vi "Teleop.vi"(10 "Match Info":T1={"Autonomous Elapsed Seconds"=0.0, "TeleOp Elapsed Seconds"=62.077, "Disabled Elapsed Seconds"=2.193, "Visited Autonomous"=FALSE, "Visited TeleOp"=TRUE, "Visited Disabled"=TRUE, "Autonomous Settings"={"Autonomous Style"=enum."Independent", "VI Refnum"=refnum}}, 11 "Call Context":T2=enum."Stop") -> ()   [LabVIEW 2016]
doc: "This VI is called for each TeleOp packet received from the DS where the robot is not disabled. It is often used to read from the joysticks and update I/O or to update setpoints for timed control loops. It should complete and return within 20 milliseconds or it may miss DS packets."
uses:
  <vilib>/Rock Robotics/WPI/DriverStation/WPI_DriverStationDerivedRobotMode.ctl
  <vilib>/Rock Robotics/WPI/DriverStation/WPI_DriverStationMatch Info.ctl
  Typedef/XBox Axis.ctl
  Typedef/XBox Buttons.ctl
  <vilib>/Rock Robotics/WPI/Solenoid/WPI_SolenoidValue.ctl
  <vilib>/Rock Robotics/WPI/Utilities/WPI_GetSetVariantRefNum.vi
  <vilib>/Rock Robotics/Network Tables/NT Write Boolean Array.vi
  <vilib>/Rock Robotics/Network Tables/NT Write Numeric Array.vi
  <vilib>/Rock Robotics/WPI/Solenoid/WPI_SolenoidSetEnum.vi
  SubSystems/Drive/Drive System.lvlib
  SubSystems/Intake/Intake.lvlib
  Vision/Vision Drive/Vision Drive.lvlib
panel:
  in  "Y Motor Deadbnd":dbl(slide)=0.5510204081632653 scale=0.0..1.0
  in  "X Motor Deadbnd":dbl(slide)=0.6836734693877551 scale=0.0..1.0
  in  "Y max power":dbl(slide)=0.7244897959183673 scale=0.0..1.0
  in  "X max power":dbl(slide)=0.6326530612244897 scale=0.0..1.0
  in  "Y sensitivity 2":dbl(slide)=1.0 scale=0.0..1.0
  in  "X sensitivity 2":dbl(slide)=0.2857142857142857 scale=0.0..1.0
  in  "X Joy Dead":dbl=0.06
  in  "Y Joy Dead":dbl=0.08
  out "Angle":dbl
  in  "Reset Gyro":bool
  in  "Value":bool
  in  "Setting":enum16{"Custom", "Boiler", "Gear"}(ring)
  in  "Custom":i32
  in  "X sensitivity":dbl(slide) scale=0.0..1.0
  in  "X deadband":dbl=0.3
  in  "Y sensitivity":dbl(slide)=1.0 scale=0.0..1.0
  in  "Y deadband":dbl=0.38
  # "Normal Mode"
  # "Climb Mode"
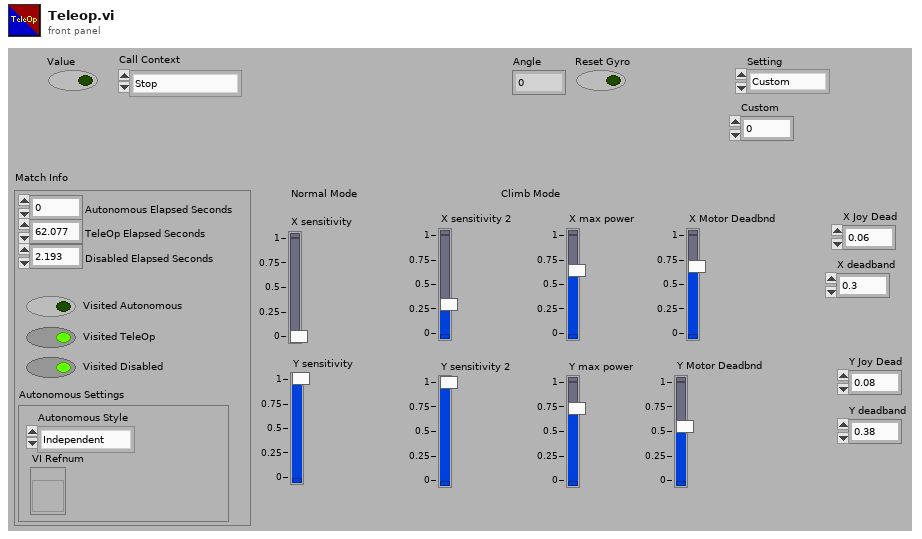
[diagram p1: front panel]
types:
  T1 = typedef "WPI_DriverStationMatch Info.ctl" = cluster{"Autonomous Elapsed Seconds":dbl, "TeleOp Elapsed Seconds":dbl, "Disabled Elapsed Seconds":dbl, "Visited Autonomous":bool, "Visited TeleOp":bool, "Visited Disabled":bool, "Autonomous Settings":cluster{"Autonomous Style":enum16{"Iterative", "Independent"}, "VI Refnum":refnum<vi>}}
  T2 = typedef "WPI_DriverStationDerivedRobotMode.ctl" = enum16{"Init", "Execute", "Stop"}
  T3 = typedef "XBox Buttons.ctl" = enum16{"A", "B", "X", "Y", "Left Bumper", "Right Bumper", "Back", "Start", "Left Joystick", "Right Joystick"}
  T4 = typedef "XBox Axis.ctl" = enum16{"Left X", "Left Y", "Left Trigger", "Right Trigger", "Right X", "Right Y"}
  T5 = typedef "WPI_JoystickDevRef.ctl" = cluster{"Device":T6}
  T6 = typedef "WPI_JoystickDeviceEnum.ctl" = enum16{"USB 0", "USB 1", "USB 2", "USB 3", "USB 4", "USB 5"}
  T7 = typedef "WPI_GyroDevRef.ctl" = cluster{"DevStatus":errorcluster, "Analog Channel":T8, "Offset":dbl, "Gain (VoltsPerDegree/Second)":dbl, "Gyro Type":enum16{"Analog", "XRS450"}, "Handle":i32, "SPI Bus":T9, "Device Found":bool, "Sample Rate":dbl, "Calibrate On Open":bool}
  T8 = typedef "FPGA_AIChannel.ctl" = enum8{"AI 0", "AI 1", "AI 2", "AI 3", "AI MXP 0", "AI MXP 1", "AI MXP 2", "AI MXP 3", "Invalid"}
  T9 = typedef "spi_bus.ctl" = enum16{"SPI On-Board, CS0", "SPI On-Board, CS1", "SPI On-Board, CS2", "SPI On-Board, CS3", "SPI MXP", "Invalid"}
  T10 = typedef "WPI_MotorControlDeviceRef.ctl" = cluster{"DeviceStatus":errorcluster, "Type":T11, "PWM":cluster{"PWM Channel":T12, "DeadBand":T13}, "CAN":cluster{"Device Number":u8, "SetOutput VI Ref":variant, "GetOutput VI Ref":variant, "Enable VI Ref":variant, "Disable VI Ref":variant, "Data":variant}, "Invert":bool}
  T11 = typedef "WPI_MotorControlType.ctl" = enum16{"PWM", "CAN"}
  T12 = typedef "FPGA_DIOPWMChannel.ctl" = enum8{"PWM 0", "PWM 1", "PWM 2", "PWM 3", "PWM 4", "PWM 5", "PWM 6", "PWM 7", "PWM 8", "PWM 9", "PWM MXP 0", "PWM MXP 1", "PWM MXP 2", "PWM MXP 3", "PWM MXP 4", "PWM MXP 5", "PWM MXP 6", "PWM MXP 7", "PWM MXP 8", "PWM MXP 9", "Invalid"}
  T13 = typedef "WPI_PWMDeadband.ctl" = cluster{"Name":string, "maxPositivePwm":i32, "minPositivePwm":i32, "centerPwm":i32, "maxNegativePwm":i32, "minNegativePwm":i32, "angularRange":u16}
  T14 = typedef "WPI_SolenoidValue.ctl" = enum16{"Off", "On", "Forward", "Reverse"}
  T15 = typedef "WPI_SolenoidDevRef.ctl" = cluster{"DevStatus":errorcluster, "Pneumatics Control Module":u8, "Forward Solenoid Channel":T16, "Reverse Solenoid Channel":T16}
  T16 = typedef "WPI_SolenoidChannel.ctl" = enum8{"Solenoid 0", "Solenoid 1", "Solenoid 2", "Solenoid 3", "Solenoid 4", "Solenoid 5", "Solenoid 6", "Solenoid 7", "Invalid"}
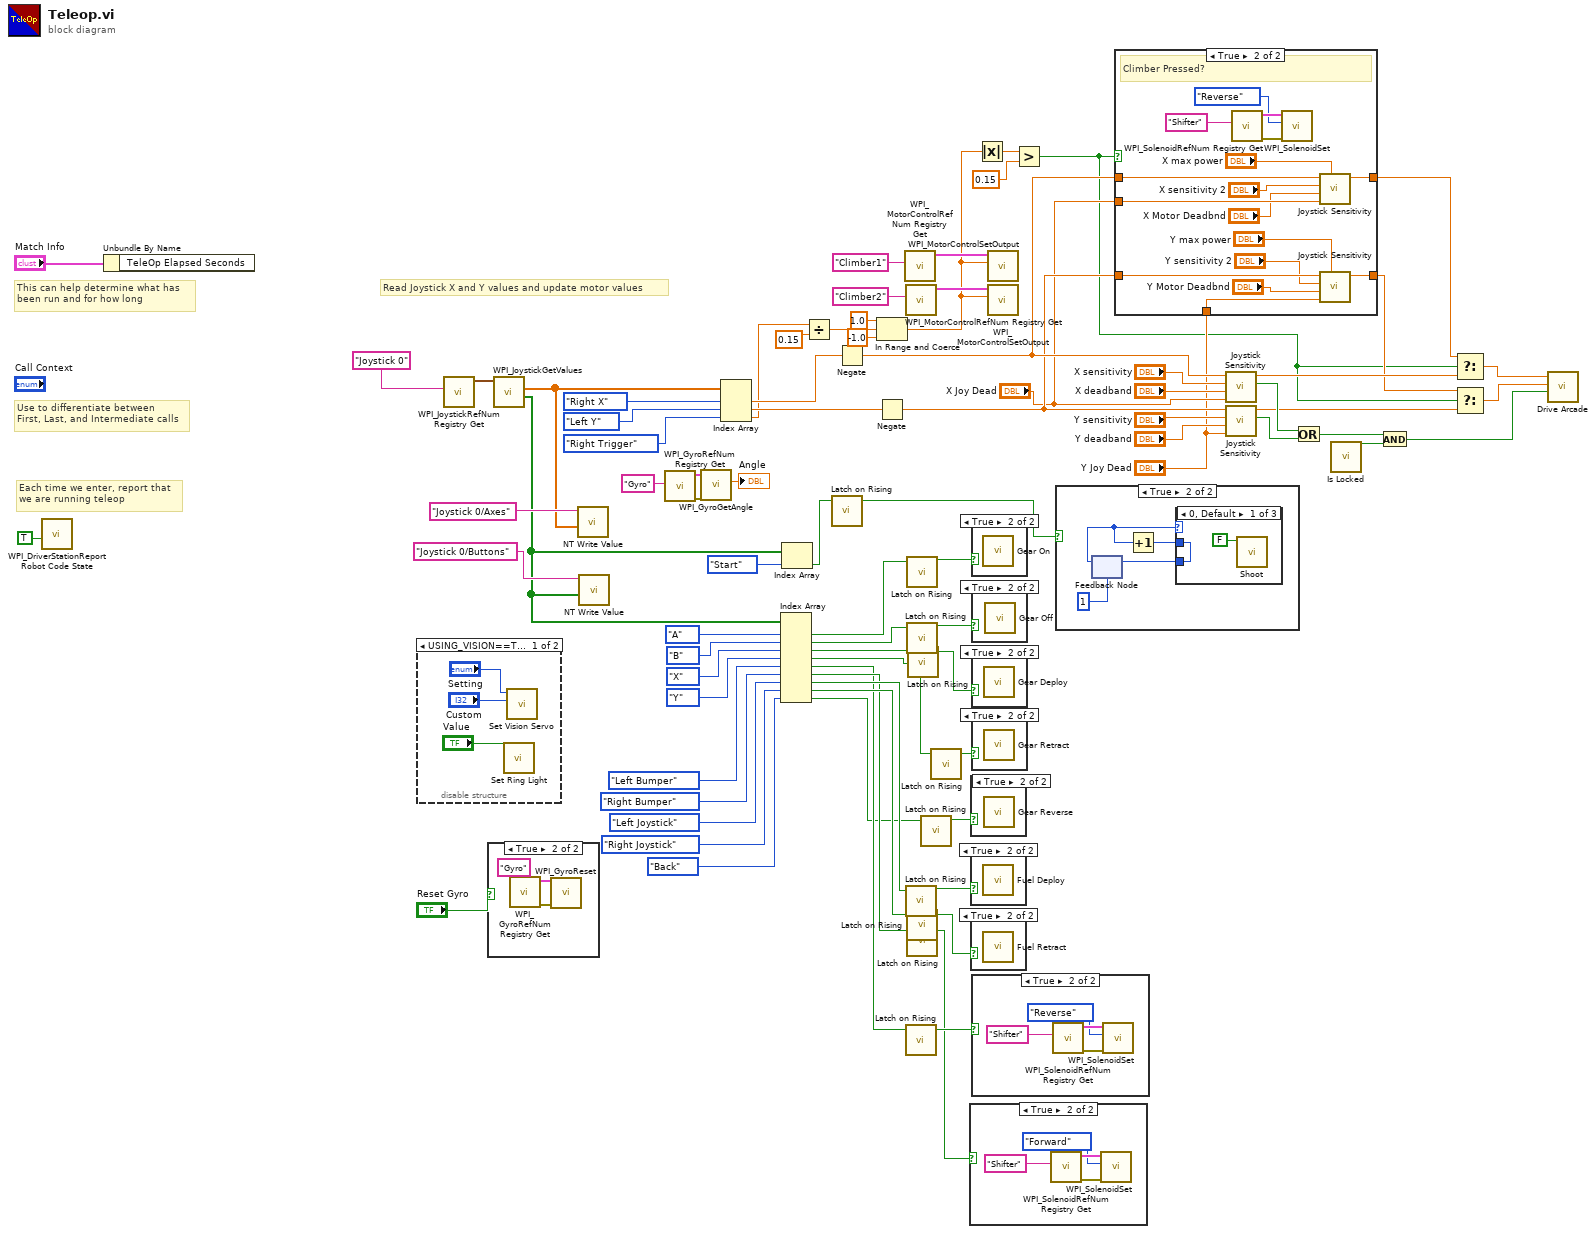
[diagram p0: block diagram]
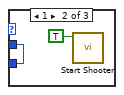
[diagram p5: hidden frame]
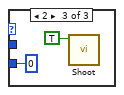
[diagram p6: hidden frame]
diagram:
  # "Each time we enter, report that\nwe are running teleop"
  # "Use to differentiate between\nFirst, Last, and Intermediate calls"
  # "This can help determine what has\nbeen run and for how long"
  # "Read Joystick X and Y values and update motor values"
  n1 = call <vilib>:"WPI_DriverStationReport Robot Code State.vi"("TeleOp"=TRUE ("Autonomous")) -> ()  [unwired: 10 in, 1 out]
  n2 = Unbundle By Name("Match Info") -> ()  [unwired: 1 out]
  n3 = disable-structure shown="USING_VISION==TRUE" {
    frame condition #0 (active) {
      n4 = call "Set Ring Light.vi"("Light On? (F)"="Value") -> ()  [unwired: 10 in, 1 out]
      n5 = call "Set Vision Servo.vi"("Custom"="Custom", "Setting"="Setting") -> ()  [unwired: 9 in, 1 out]
    }
    frame condition #1 {
    }
  }
  n6 = call <vilib>:"WPI_JoystickRefNum Registry Get.vi"("refnum name"="Joystick 0") -> ("JoystickDevRef"=w78:T5)  [unwired: 1 in, 9 out]
  n7 = case shown="True" "Reset Gyro" {
    frame False {
    }
    frame True {
      n8 = call <vilib>:"WPI_GyroRefNum Registry Get.vi"("refnum name"="Gyro") -> ("error out"=w86:errorcluster, "GyroDevRef"=w85:T7)  [unwired: 9 in]
      n9 = call <vilib>:"WPI_GyroReset.vi"("error in"=w86, "GyroDevRef"=w85) -> ()  [unwired: 8 in, 2 out]
    }
  }
  n10 = call <vilib>:"WPI_JoystickGetValues.vi"("JoystickDevRef"=w78) -> ("Buttons"=w33:bool[], "Axes"=w74:dbl[])  [unwired: 6 in, 3 out]
  n11 = call-poly <vilib>:"NT Write Value.vi"("Numeric Array"=w74, "Name"="Joystick 0/Axes") -> ()  [unwired: 9 in, 1 out]
  n12 = call-poly <vilib>:"NT Write Value.vi"("Boolean Array"=w33, "Name"="Joystick 0/Buttons") -> ()  [unwired: 9 in, 1 out]
  n13 = call <vilib>:"WPI_GyroRefNum Registry Get.vi"("refnum name"="Gyro") -> ("error out"=w28:errorcluster, "GyroDevRef"=w27:T7)  [unwired: 9 in]
  n14 = call <vilib>:"WPI_GyroGetAngle.vi"("error in"=w28, "GyroDevRef"=w27) -> ("Angle"=→"Angle":dbl)  [unwired: 5 in, 4 out]
  n15 = Index Array(array=w74, index #1=XBox_Axis."Right X" ("Enum"), index #2=XBox_Axis."Left Y" ("Enum"), index #3=XBox_Axis."Right Trigger" ("Enum")) -> (element #1=w48:dbl, element #2=w71:dbl, element #3=w37:dbl)
  n16 = Index Array(array=w33, index #1=XBox_Buttons."A" ("Enum"), index #2=XBox_Buttons."B" ("Enum"), index #3=XBox_Buttons."X" ("Enum"), index #4=XBox_Buttons."Y" ("Enum"), index #5=XBox_Buttons."Left Bumper" ("Enum"), index #6=XBox_Buttons."Right Bumper" ("Enum"), index #7=XBox_Buttons."Left Joystick" ("Enum"), index #8=XBox_Buttons."Right Joystick" ("Enum"), index #9=XBox_Buttons."Back" ("Enum")) -> (element #1=w62:bool, element #2=w59:bool, element #3=w57:bool, element #4=w49:bool, element #5=w51:bool, element #6=w52:bool, element #7=w54:bool, element #8=w53:bool, element #9=w1:bool)
  n17 = Index Array(array=w33, index=XBox_Buttons."Start" ("Enum")) -> (element=w31:bool)
  n18 = Divide(x=w37, y=0.15 ("x")) -> (x/y=w20:dbl)
  n19 = call "Latch on Rising.vi"("Boolean in"=w31) -> ("Boolean out"=w16:bool)  [unwired: 4 in]
  n20 = Negate(x=w48) -> (-x=w11:dbl)
  n21 = In Range and Coerce(upper limit=1.0, x=w20, lower limit=-1.0) -> (coerced(x)=w15:dbl)  [unwired: 1 out]
  n22 = Negate(x=w71) -> (-x=w10:dbl)
  n23 = call <vilib>:"WPI_MotorControlRefNum Registry Get.vi"("refnum name"="Climber1") -> ("MotorControlDevRef"=w38:T10)  [unwired: 9 in, 1 out]
  n24 = call <vilib>:"WPI_MotorControlRefNum Registry Get.vi"("refnum name"="Climber2") -> ("MotorControlDevRef"=w39:T10)  [unwired: 9 in, 1 out]
  n25 = call "Latch on Rising.vi"("Boolean in"=w54) -> ("Boolean out"=w55:bool)  [unwired: 4 in]
  n26 = call "Latch on Rising.vi"("Boolean in"=w51) -> ("Boolean out"=w43:bool)  [unwired: 4 in]
  n27 = call "Latch on Rising.vi"("Boolean in"=w62) -> ("Boolean out"=w61:bool)  [unwired: 4 in]
  n28 = call "Latch on Rising.vi"("Boolean in"=w59) -> ("Boolean out"=w60:bool)  [unwired: 4 in]
  n29 = call "Latch on Rising.vi"("Boolean in"=w53) -> ("Boolean out"=w56:bool)  [unwired: 4 in]
  n30 = call "Latch on Rising.vi"("Boolean in"=w52) -> ("Boolean out"=w42:bool)  [unwired: 4 in]
  n31 = call "Latch on Rising.vi"("Boolean in"=w57) -> ("Boolean out"=w58:bool)  [unwired: 4 in]
  n32 = call "Latch on Rising.vi"("Boolean in"=w1) -> ("Boolean out"=w2:bool)  [unwired: 4 in]
  n33 = call "Latch on Rising.vi"("Boolean in"=w49) -> ("Boolean out"=w50:bool)  [unwired: 4 in]
  n34 = case shown="True" w42 {
    frame False {
    }
    frame True {
      n35 = call <vilib>:"WPI_SolenoidRefNum Registry Get.vi"("refnum name"="Shifter") -> ("error out"=w89:errorcluster, "SolenoidDevRef"=w88:T15)  [unwired: 9 in]
      n36 = call-poly <vilib>:"WPI_SolenoidSet.vi"("error in (no error)"=w89, "Value"=WPI_SolenoidValue."Forward", "SolenoidDevRef"=w88) -> ()  [unwired: 7 in, 2 out]
    }
  }
  n37 = case shown="True" w2 {
    frame False {
    }
    frame True {
      n38 = call "Gear Reverse.vi"() -> ()  [unwired: 11 in, 1 out]
    }
  }
  n39 = case shown="True" w55 {
    frame False {
    }
    frame True {
      n40 = call "Fuel Deploy.vi"() -> ()  [unwired: 11 in, 1 out]
    }
  }
  n41 = case shown="True" w56 {
    frame False {
    }
    frame True {
      n42 = call "Fuel Retract.vi"() -> ()  [unwired: 11 in, 1 out]
    }
  }
  n43 = case shown="True" w61 {
    frame False {
    }
    frame True {
      n44 = call "Gear On.vi"() -> ()  [unwired: 11 in, 1 out]
    }
  }
  n45 = case shown="True" w60 {
    frame False {
    }
    frame True {
      n46 = call "Gear Off.vi"() -> ()  [unwired: 11 in, 1 out]
    }
  }
  n47 = case shown="True" w58 {
    frame False {
    }
    frame True {
      n48 = call "Gear Deploy.vi"() -> ()  [unwired: 11 in, 1 out]
    }
  }
  n49 = case shown="True" w50 {
    frame False {
    }
    frame True {
      n50 = call "Gear Retract.vi"() -> ()  [unwired: 11 in, 1 out]
    }
  }
  n51 = case shown="True" w43 {
    frame False {
    }
    frame True {
      n52 = call <vilib>:"WPI_SolenoidRefNum Registry Get.vi"("refnum name"="Shifter") -> ("error out"=w93:errorcluster, "SolenoidDevRef"=w92:T15)  [unwired: 9 in]
      n53 = call-poly <vilib>:"WPI_SolenoidSet.vi"("error in (no error)"=w93, "Value"=WPI_SolenoidValue."Reverse", "SolenoidDevRef"=w92) -> ()  [unwired: 7 in, 2 out]
    }
  }
  n54 = Absolute Value(x=w15) -> (abs(x)=w5:dbl)
  n55 = call <vilib>:"WPI_MotorControlSetOutput.vi"("Output"=w15, "MotorControlDevRef"=w38) -> ()  [unwired: 7 in, 3 out]
  n56 = call <vilib>:"WPI_MotorControlSetOutput.vi"("Output"=w15, "MotorControlDevRef"=w39) -> ()  [unwired: 7 in, 3 out]
  n57 = Greater?(x=w5, y=0.15) -> (0:w4:bool)
  n58 = case shown="True" w16 {
    frame False {
    }
    frame True {
      n59 = feedback #1(1) -> (w97:i32)
      n60 = Increment(x=w97) -> (x+1=w96:i32)
      n61 = case shown="0, Default" w97 {
        tunnel: w96 -> [w99 w101 _]
        tunnel: [w99 w101 0] -> w95
        frame 0, Default {
          n62 = call "Shoot.vi"("Enabled? (F)"=FALSE) -> ()  [unwired: 10 in, 1 out]
        }
        frame 1 {
          n63 = call "Start Shooter.vi"("Enabled? (F)"=TRUE) -> ()  [unwired: 10 in, 1 out]
        }
        frame 2 {
          n64 = call "Shoot.vi"("Enabled? (F)"=TRUE) -> ()  [unwired: 10 in, 1 out]
        }
      }
      n65 = feedback-in #1(w95) -> ()
    }
  }
  n66 = case shown="True" w4 {
    tunnel: w11 -> [w105 w118]
    tunnel: w10 -> [w106 w117]
    tunnel: [w105 w116] -> w8
    tunnel: [w106 w115] -> w9
    tunnel: "X Joy Dead" -> [_ w113]
    tunnel: "Y Joy Dead" -> [_ w112]
    frame False {
    }
    frame True {
      # "Climber Pressed?"
      n67 = call <vilib>:"WPI_SolenoidRefNum Registry Get.vi"("refnum name"="Shifter") -> ("error out"=w121:errorcluster, "SolenoidDevRef"=w120:T15)  [unwired: 9 in]
      n68 = call-poly <vilib>:"WPI_SolenoidSet.vi"("error in (no error)"=w121, "Value"=WPI_SolenoidValue."Reverse", "SolenoidDevRef"=w120) -> ()  [unwired: 7 in, 2 out]
      n69 = call "Joystick Sensitivity.vi"("max power (1)"="X max power", "joystick deadband"=w113, "motor deadband (0.15)"="X Motor Deadbnd", "sensitivity (0.5)"="X sensitivity 2", "x"=w118) -> ("y"=w116:dbl)  [unwired: 5 in, 1 out]
      n70 = call "Joystick Sensitivity.vi"("max power (1)"="Y max power", "joystick deadband"=w112, "motor deadband (0.15)"="Y Motor Deadbnd", "sensitivity (0.5)"="Y sensitivity 2", "x"=w117) -> ("y"=w115:dbl)  [unwired: 5 in, 1 out]
    }
  }
  n71 = call "Joystick Sensitivity.vi"("joystick deadband"="X Joy Dead", "motor deadband (0.15)"="X deadband", "sensitivity (0.5)"="X sensitivity", "x"=w11) -> ("Outside Deadband?"=w35:bool, "y"=w25:dbl)  [unwired: 6 in]
  n72 = call "Joystick Sensitivity.vi"("joystick deadband"="Y Joy Dead", "motor deadband (0.15)"="Y deadband", "sensitivity (0.5)"="Y sensitivity", "x"=w10) -> ("Outside Deadband?"=w34:bool, "y"=w24:dbl)  [unwired: 6 in]
  n73 = Or(x=w35, y=w34) -> (x .or. y?=w23:bool)
  n74 = call "Is Locked.vi"() -> ("Locked?"=w22:bool)  [unwired: 10 in, 1 out]
  n75 = And(x=w23, y=w22) -> (x .and. y?=w21:bool)
  n76 = Select(t=w8, s=w4, f=w25) -> (s? t:f=w13:dbl)
  n77 = Select(t=w9, s=w4, f=w24) -> (s? t:f=w12:dbl)
  n78 = call "Drive Arcade.vi"("Force? (F)"=w21, "Y Axis"=w12, "X Axis"=w13) -> ()  [unwired: 8 in, 1 out]
